vi "ConfigureTrigger.vi"(0 "object in":refnum<class "AD2_MSO_SDK.lvclass">, 5 "error in (no error)":errorcluster) -> (14 "object out":refnum<class "AD2_MSO_SDK.lvclass">, 19 "error out":errorcluster)   [LabVIEW 2019, in "AD2_MSO_SDK.lvclass"]
uses:
  AD2_MSO_SDK.lvclass
  AD2_MSO_SDK.lvclass/AD2_MSO_SDK.ctl
  Olasdwf/Olasdwf.lvlib
panel:
  in  "Trigger Mode":u16(ring) items=["None", "Auto", "Normal"]
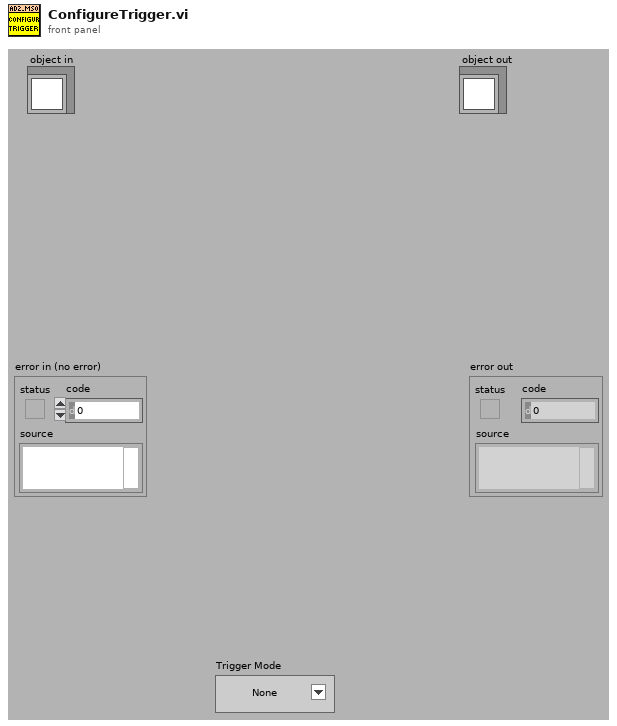
[diagram p1: front panel]
types:
  T1 = typedef "AD2_MSO_SDK.lvclass/AD2TriggerSources.ctl" = enum8{"trigrsrcNone", "trigsrcPC", "trigsrcDetectorAnalogIn", "trigsrcDetectorDigitalIn", "trigsrcAnalogIn", "trigsrcDigitalIn", "trigsrcDigitalOut", "trigsrcAnalogOut1", "trigsrcAnalogOut2", "trigsrcAnalogOut3", "trigsrcAnalogOut4", "trigsrcExternal1", "trigsrcExternal2", "trigsrcExternal3", "trigsrcExternal4", ""}
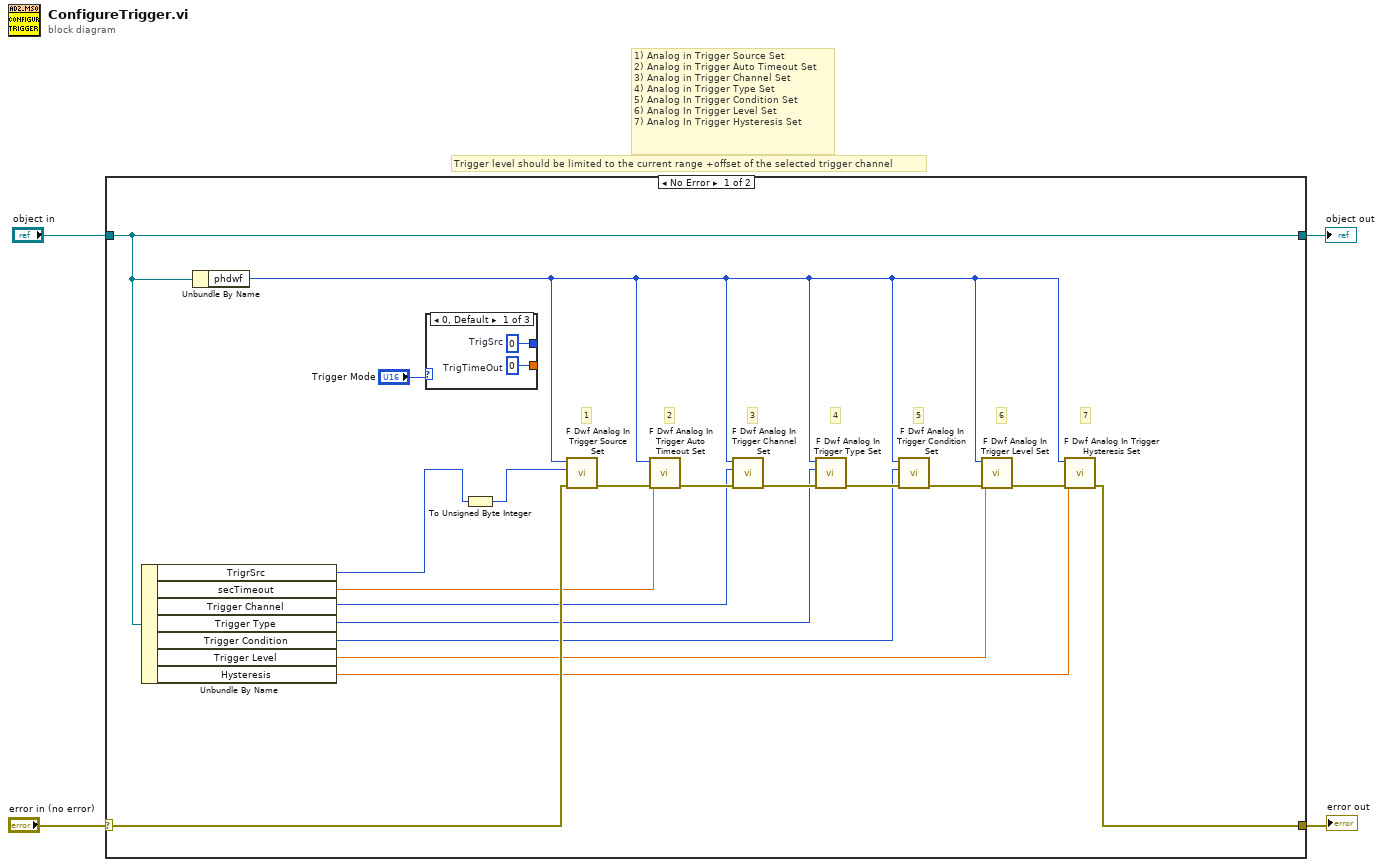
[diagram p0: block diagram]
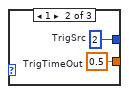
[diagram p2: hidden frame]
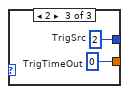
[diagram p3: hidden frame]
diagram:
  # "Trigger level should be limited to the current range +offset of the selected trigger channel"
  # "1) Analog in Trigger Source Set\n2) Analog in Trigger Auto Timeout Set\n3) Analog in Trigger Channel Set\n4) Analog in Trigger Type Set\n5) Analog In Trigger Condition Set\n6) Analog In Trigger Level Set\n7) Analog In Trigger Hysteresis Set"
  n1 = case shown="No Error" "error in (no error)" {
    selector: "error in (no error)" -> [w15 w31]
    tunnel: [w14 w31] -> w3
    tunnel: [w12 w30] -> w1
    tunnel: "object in" -> [w12 w30]
    frame No Error {
      # "7"
      # "6"
      # "5"
      # "4"
      # "3"
      # "2"
      # "1"
      n2 = Unbundle By Name(w12) -> ("TrigrSrc"=w5:T1, "secTimeout"=w11:dbl, "Trigger Channel"=w10:i32, "Trigger Type"=w9:i32, "Trigger Condition"=w8:i32, "Trigger Level"=w7:dbl, "Hysteresis"=w6:dbl)
      n3 = Unbundle By Name(w12) -> ("phdwf"=w16:i32)
      n4 = case shown="0, Default" "Trigger Mode" {
        tunnel: [w25 w27 w29] -> _
        tunnel: [w24 w26 w28] -> _
        frame 0, Default {
          w24 = 0  # TrigTimeOut
          w25 = u8 0  # TrigSrc
        }
        frame 1 {
          w26 = 0.5  # TrigTimeOut
          w27 = u8 2  # TrigSrc
        }
        frame 2 {
          w28 = 0  # TrigTimeOut
          w29 = u8 2  # TrigSrc
        }
      }
      n5 = To Unsigned Byte Integer(number=w5) -> (unsigned 8bit integer=w13:u8)
      n6 = call "F Dwf Analog In Trigger Source Set.vi"("error in (no error)"=w15, "trigsrc"=w13, "hdwf"=w16) -> ("error out"=w22:errorcluster)  [unwired: 7 in, 1 out]
      n7 = call "F Dwf Analog In Trigger Auto Timeout Set.vi"("error in (no error)"=w22, "secTimeout"=w11, "hdwf"=w16) -> ("error out"=w21:errorcluster)  [unwired: 7 in, 1 out]
      n8 = call "F Dwf Analog In Trigger Channel Set.vi"("error in (no error)"=w21, "idxChannel"=w10, "hdwf"=w16) -> ("error out"=w20:errorcluster)  [unwired: 7 in, 1 out]
      n9 = call "F Dwf Analog In Trigger Type Set.vi"("error in (no error)"=w20, "trigtype"=w9, "hdwf"=w16) -> ("error out"=w19:errorcluster)  [unwired: 7 in, 1 out]
      n10 = call "F Dwf Analog In Trigger Condition Set.vi"("error in (no error)"=w19, "trigcond"=w8, "hdwf"=w16) -> ("error out"=w18:errorcluster)  [unwired: 7 in, 1 out]
      n11 = call "F Dwf Analog In Trigger Level Set.vi"("error in (no error)"=w18, "voltsLevel"=w7, "hdwf"=w16) -> ("error out"=w17:errorcluster)  [unwired: 7 in, 1 out]
      n12 = call "F Dwf Analog In Trigger Hysteresis Set.vi"("error in (no error)"=w17, "voltsLevel"=w6, "hdwf"=w16) -> ("error out"=w14:errorcluster)  [unwired: 7 in, 1 out]
    }
    frame Error {
    }
  }
  "error out" <- w3
  "object out" <- w1
